vi "Hardware-Skipfire.vi"(8 "error in (no error)":errorcluster, 11 "DCM-DSI in":refnum<class "DCM-DSI.lvclass">) -> (0 "error out":errorcluster, 3 "DCM-DSI out":refnum<class "DCM-DSI.lvclass">)   [LabVIEW 2016, in "DSI-RT.lvlib"]
uses:
  DSI-RT.lvlib
  Classes/DCM-DSI/DCM-DSI.lvclass
  Classes/DCM-DSI/Read DCM Ref.vi
  Classes/DCM-DSI/Read Skip Fire Setup.vi
  Classes/DCM-DSI/Write Skip Fire Setup.vi
  <vilib>/Powertrain Controls/Device Drivers/DCM/Rev0/RT/DCM - RT.lvclass
  <vilib>/Powertrain Controls/Device Drivers/DCM/Skip Fire/RT/DCM - RT - Skip Fire.lvlib
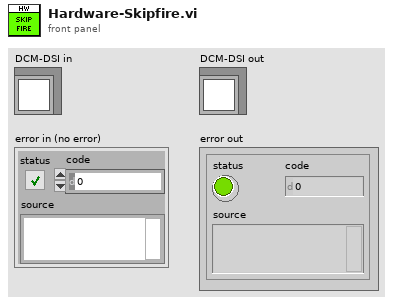
[diagram p1: front panel]
types:
  T1 = typedef "DCM - RT - Skip Fire.lvlib/Skip Fire Setup.ctl" = cluster{"Enable":bool, "Total Cycles":u8, "On Cycles":u8, "TDC Offset [CAD]":sgl}
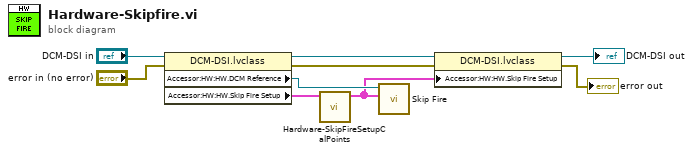
[diagram p0: block diagram]
diagram:
  n1 = property class="DCM-DSI.lvclass"(reference="DCM-DSI in", error in="error in (no error)") -> (reference out=w5:refnum<class "DCM-DSI.lvclass">, error out=w6:errorcluster, "Accessor:HW:HW.DCM Reference"=w9:refnum<class "DCM - RT.lvclass">, "Accessor:HW:HW.Skip Fire Setup"=w2:T1[])
  n2 = call "Hardware-SkipFireSetupCalPoints.vi"("Skipfire Setup"=w2) -> ("Skipfire Setup"=w4:T1[])  [unwired: 10 in]
  n3 = call <vilib>:"Skip Fire.vi"("Skip Fire Setup"=w4, "DCM Reference"=w9) -> ()  [unwired: 10 in]
  n4 = property class="DCM-DSI.lvclass"(reference=w5, error in=w6, "Accessor:HW:HW.Skip Fire Setup"=w4) -> (reference out=→"DCM-DSI out":refnum<class "DCM-DSI.lvclass">, error out=→"error out":errorcluster)
